vi "Do.vi"(8 "error in":errorcluster, 10 "Actor in":refnum<class "Actor.lvclass">, 11 "Update Fan Voltage MSG":refnum<class "Update Fan Voltage MSG.lvclass">) -> (0 "error out":errorcluster, 2 "Actor out":refnum<class "Actor.lvclass">)   [LabVIEW 2017, in "Controller.lvlib" / "Update Fan Voltage MSG.lvclass"]
doc: "(<B>Filename</B>: Actor Framework.lvlib:Message.lvclass:Do.vi)\n\nDefines what a message does when it is received by an actor. Generally, a message instructs an actor to invoke one of its methods. By default, this method does nothing. A child class must override it to define behavior. Create a child class by using the Actor Framework Message Maker dialog box."
uses:
  Update Fan Voltage MSG.lvclass
  <vilib>/ActorFramework/Actor/Actor.lvclass
  gController.lvclass
  Update Fan Voltage MSG.lvclass/Update Fan Voltage MSG.ctl
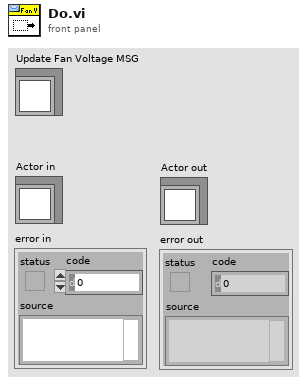
[diagram p1: front panel]
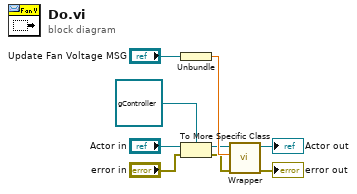
[diagram p0: block diagram]
diagram:
  n1 = Unbundle("Update Fan Voltage MSG") -> (w4:dbl)
  n2 = To More Specific Class(target class=refnum<class "gController.lvclass"> refnum ("Controller.lvlib:gController"), reference="Actor in", error in="error in") -> (specific class reference=w2:refnum<class "gController.lvclass">, error out=w1:errorcluster)
  n3 = call "Wrapper.vi"("error in"=w1, "Voltage"=w4, "gController in"=w2) -> ("error out"=→"error out":errorcluster, "Actor out"=→"Actor out":refnum<class "Actor.lvclass">)  [unwired: 7 in]
